vi "Common_Test_Template.vi"() -> ()   [LabVIEW 2013]
uses:
  Controls/USID.ctl
  <vilib>/NI_TestStand_SemiconductorModule/NI_TestStand_Semiconductor_Module.lvlibp/PinMap/General/SemiconductorModuleContext.ctl
  <vilib>/NI_TestStand_SemiconductorModule/NI_TestStand_Semiconductor_Module.lvlibp
panel:
  in  "Semiconductor Module Context":T1
  in  "All_Scripts":string[][](array[string])
  in  "Pins":string[](array[string])=["CLK", "SDA"]
  in  "USID":T2 max=15
  in  "Test Name":string="IVIOKGD"
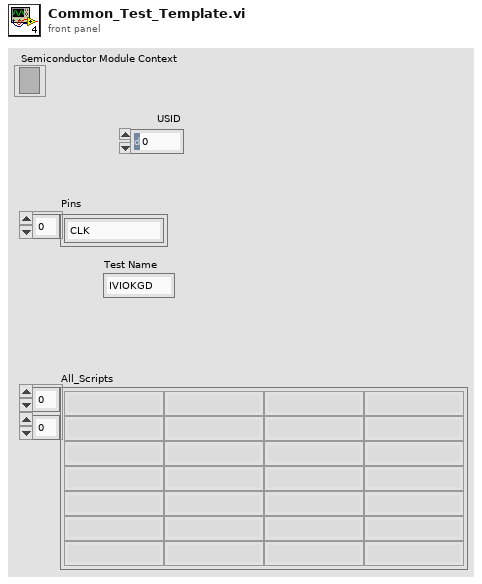
[diagram p1: front panel]
types:
  T1 = typedef "NI_TestStand_Semiconductor_Module.lvlibp/SemiconductorModuleContext.ctl" = refnum<k7>
  T2 = typedef "USID.ctl" = u8
  T3 = typedef "Reg_Address_Data.ctl" = cluster{"Address":u8, "Data":u8}
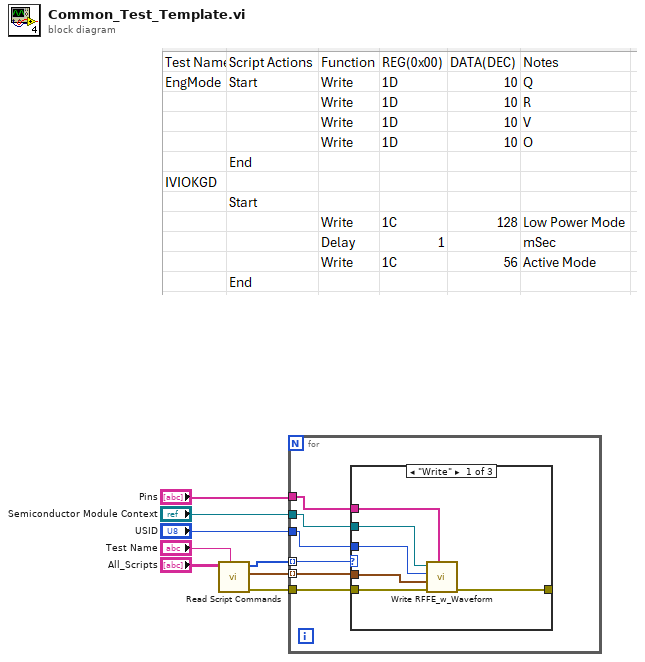
[diagram p0: block diagram]
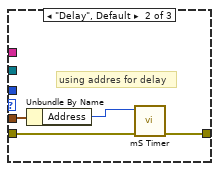
[diagram p2: hidden frame]
diagram:
  n1 = call "Read Script Commands.vi"("Test Name"="Test Name", "All_Scripts"="All_Scripts") -> ("Error Out"=w3:errorcluster, "Script_Data"=w4:T3[], "Script_Functions"=w5:enum16{"Write", "Delay", "Read"}[])  [unwired: 7 in]
  n2 = for {
    tunnel: "USID" -> [w11]
    tunnel: w5 -> [w14] mode=indexing
    tunnel: w4 -> [w13] mode=indexing
    tunnel: w3 -> [w12]
    tunnel: "Semiconductor Module Context" -> [w10]
    tunnel: "Pins" -> [w9]
    n3 = case shown="\"Write\"" w14 {
      tunnel: w13 -> [w17 w23 _]
      tunnel: w12 -> [w20 w24 w25]
      tunnel: w11 -> [w19 _ _]
      tunnel: w10 -> [w18 _ _]
      tunnel: w9 -> [w16 _ _]
      tunnel: [w15 w21 w25] -> _
      frame "Write" {
        n4 = call "Write RFFE_w_Waveform.vi"("Pins"=w16, "error in (no error)"=w20, "Reg_Address_Data"=w17, "USID"=w19, "Semiconductor Module Context"=w18) -> ("error out"=w15:errorcluster)  [unwired: 5 in, 1 out]
      }
      frame "Delay", Default {
        # "using addres for delay"
        n5 = Unbundle By Name(w23) -> ("Address"=w22:u8)
        n6 = call "mS Timer.vi"("Error In"=w24, "Delay(S)"=w22) -> ("Error Out"=w21:errorcluster)  [unwired: 9 in]
      }
      frame "Read" {
      }
    }
  }
